vi "SOUR_POW_CORR_COLL_DISP_STAT.vi"(0 "VISA IN":refnum<visa-resource-name>, 1 "Display ON/OFF":bool, 5 "error in":errorcluster, 7 "Channel":i32) -> (14 "VISA Out":refnum<visa-resource-name>, 19 "error out":errorcluster)   [LabVIEW 2018, in "PNA-X.lvlib"]
doc: "SOURce<cnum>:POWer:CORRection:COLLect:DISPlay[:STATe] <ON | OFF> \n(Read-Write) Enables and disables the display of power readings on the PNA screen. Send this \ncommand BEFORE you begin a source power cal acquisition. After the source power cal data is \nacquired, this setting is reset to ON. \nParameters \n<cnum> Any existing channel number. If unspecified, value is set to 1 \n<ON|OFF> ON (1) Source power calibration dialog box is shown on the PNA screen. \nPower readings are plotted against the Tolerance value as limit lines. \nOFF (0) - Source power calibration dialog box is NOT shown on the PNA \nscreen. \nExamples SOUR:POW:CORR:COLL:DISP ON \nsource1:power2:correction:collect:display:state off \nQuery Syntax SOURce:POWer:CORRection:COLLect:DISPlay[:STATe]? \nReturn Type Boolean (1 = ON, 0 = OFF) \nDefault ON (1)"
uses:
  PNA-X.lvlib
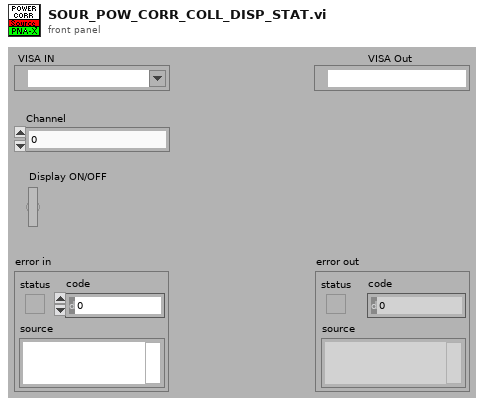
[diagram p1: front panel]
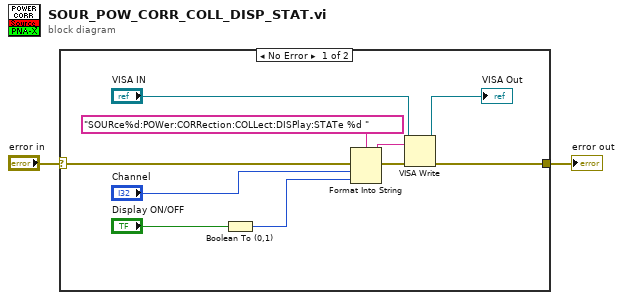
[diagram p0: block diagram]
diagram:
  n1 = case shown="No Error" "error in" {
    selector: "error in" -> [w12 w13]
    tunnel: [w7 w13] -> w1
    frame No Error {
      n2 = Boolean To (0,1)(Boolean="Display ON/OFF") -> (0, 1=w3:i16)
      n3 = Format Into String(format string="SOURce%d:POWer:CORRection:COLLect:DISPlay:STATe %d " ("Cmdline"), error in=w12, "Channel", w3) -> (resulting string=w10:string, error out=w11:errorcluster)  [unwired: 1 in]
      n4 = VISA Write(VISA resource name="VISA IN", write buffer=w10, error in (no error)=w11) -> (VISA resource name out=→"VISA Out":refnum<visa-resource-name>, error out=w7:errorcluster)  [unwired: 1 out]
    }
    frame Error {
    }
  }
  "error out" <- w1
